vi "Notify_GServer.vi"(8 "error in (no error)":errorcluster, 11 "FAMM in":refnum<class "FAMM.lvclass">) -> (0 "error out":errorcluster, 3 "FAMM out":refnum<class "FAMM.lvclass">)   [LabVIEW 2020, in "FAMM.lvclass"]
doc: "Notify the Gserver that the FAMM constructor is finished and send the Attributes reference"
uses:
  FAMM.lvclass
  Gserver/controls/Typedef_QueryType.ctl
  Gserver/controls/Typedef_Gviewer-Query.ctl
  FAMM.lvclass/FAMM.ctl
  Gserver/Gserver.lvclass
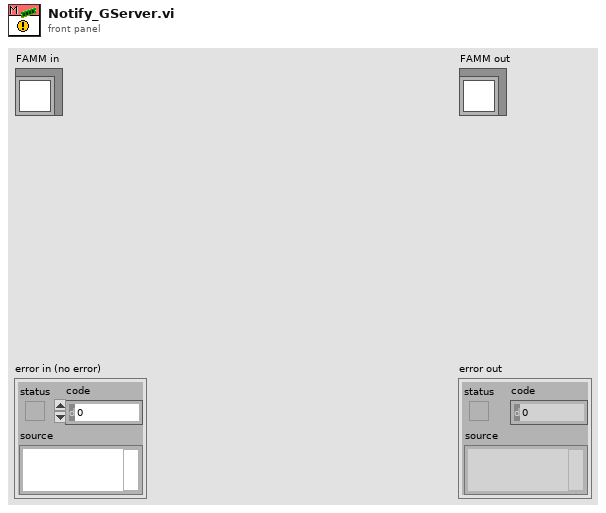
[diagram p1: front panel]
types:
  T1 = typedef "Gserver.lvclass/Typedef_QueryType.ctl" = enum16{"Subscribe", "DataRequest", "RequestAllTags", "RequestIniPath", "FAMMstarted", "SetClientOptions", "OpenNewGraph", "CloseClient", "CloseAllClients", "Close Gserver"}
  T2 = typedef "Gserver.lvclass/Typedef_Gviewer-Query.ctl" = cluster{"Query_type":T1, "data":variant, "Source":string, "Time Stamp":timestamp}
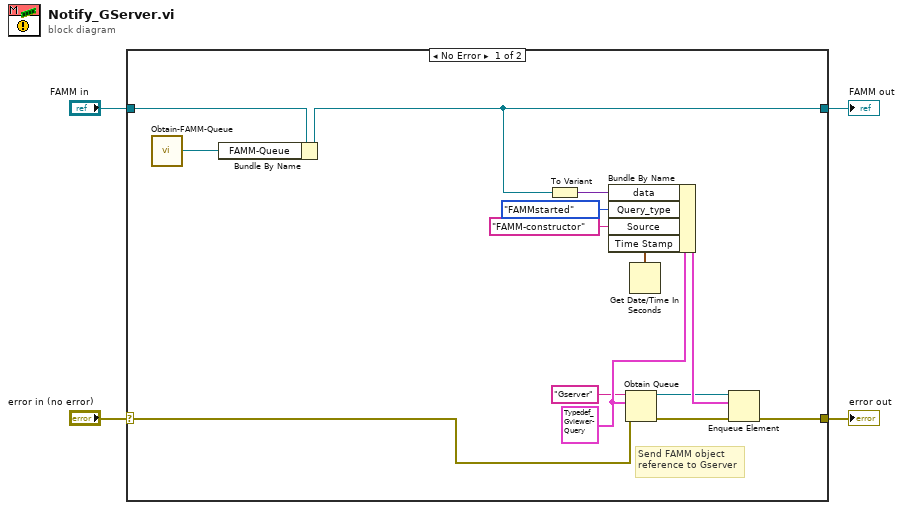
[diagram p0: block diagram]
diagram:
  n1 = case shown="No Error" "error in (no error)" {
    selector: "error in (no error)" -> [w8 w20]
    tunnel: [w9 w20] -> w3
    tunnel: [w5 w19] -> w1
    tunnel: "FAMM in" -> [w6 w19]
    frame No Error {
      w13 = T2 {"Query_type"=enum."DataRequest", "data"=variant, "Source"="", "Time Stamp"=timestamp(0 s since 1904-01-01)} ("Query")
      # "Send FAMM object\nreference to Gserver"
      n2 = call "Obtain-FAMM-Queue.vi"() -> ("FAMM-Queue"=w7:refnum<queue>)  [unwired: 7 in]
      n3 = Bundle By Name(cluster=w6, "FAMM-Queue"=w7) -> (w5:refnum<class "FAMM.lvclass">)
      n4 = To Variant(anything=w5) -> (Variant=w18:variant)
      n5 = Obtain Queue(name (unnamed)="Gserver", element data type=w13, error in (no error)=w8) -> (queue out=w12:refnum<queue>, error out=w11:errorcluster)  [unwired: 2 in, 1 out]
      n6 = Get Date/Time In Seconds() -> (seconds since 1Jan1904=w15:timestamp)
      n7 = Bundle By Name(cluster=w13, "data"=w18, "Query_type"=Typedef_QueryType."FAMMstarted", "Source"="FAMM-constructor", "Time Stamp"=w15) -> (w14:T2)
      n8 = Enqueue Element(queue=w12, element=w14, error in (no error)=w11) -> (error out=w9:errorcluster)  [unwired: 1 in, 2 out]
    }
    frame Error {
    }
  }
  "error out" <- w3
  "FAMM out" <- w1
